vi "Remote Client Metrics subVI.vi"(9 "Message size":i32=1000000, 10 "Number of Messages":i32=20, 11 "RC Type":T1=enum."STM") -> (0 "<time/message (ms)>":i32=210, 1 "bytes/second":dbl=37611866.47860837, 2 "messages/second":dbl=4.701457451810062, 3 "<size>":i32=8000044)   [LabVIEW 2019]
uses:
  lvsrc/SMOs/RemoteControl/RemoteControl.lvclass
  lvsrc/SMOs/RemoteControl/Typedefs/RC Com Type--enum.ctl
panel:
  out "length":i32=8000004
  in  "stop":bool
  out "error out":errorcluster
  out "Data out":variant
  out "Command out":string="Command1"
  in  "Command":string="Command1"
  in  "address":string
  in  "Port":u16=6341
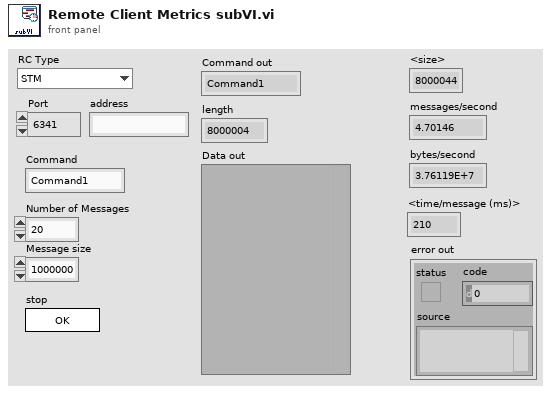
[diagram p1: front panel]
types:
  T1 = typedef "RemoteControl.lvclass/RC Com Type--enum.ctl" = enum16{"RC", "STM", "ZMQ"}
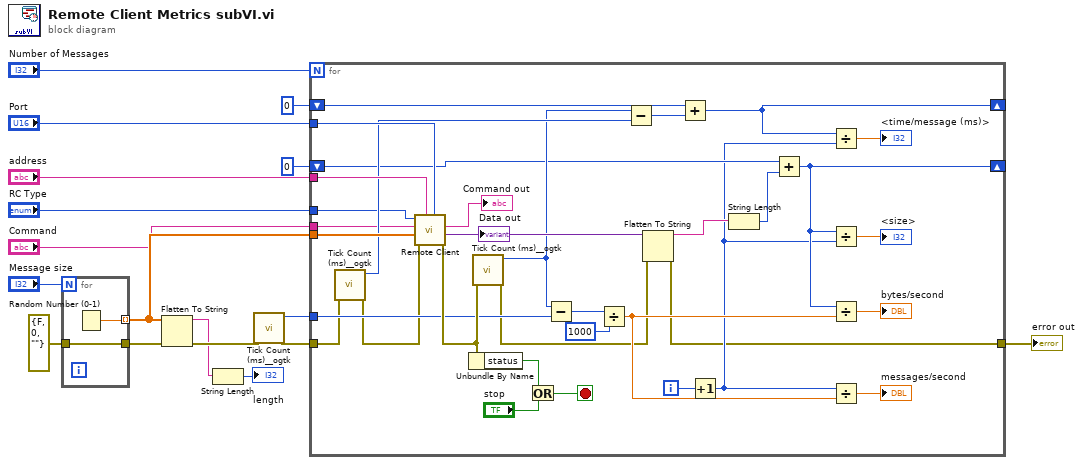
[diagram p0: block diagram]
diagram:
  n1 = for {
    N: "Message size" -> [_]
    tunnel: [w19] -> w10
    tunnel: errorcluster {"status"=FALSE, "code"=0, "source"=""} ("error in (no error)") -> [w19]
    tunnel: [w18] -> w2 mode=indexing
    n2 = Random Number (0-1)() -> (number: 0 to 1=w18:dbl)
  }
  n3 = Flatten To String(anything=w2, error in (no error)=w10) -> (data string=w7:string, error out=w9:errorcluster)  [unwired: 2 in, 1 out]
  n4 = String Length(string=w7) -> (length=→"length":i32)
  n5 = call <userlib>:"Tick Count (ms)__ogtk.vi"("error in (no error)"=w9) -> ("error out"=w14:errorcluster, "millisecond timer value"=w13:u32)  [unwired: 9 in]
  n6 = for {
    N: "Number of Messages" -> [_]
    tunnel: "Port" -> [w53]
    tunnel: [w22] -> w15
    tunnel: "address" -> [w52]
    tunnel: w14 -> [w35]
    tunnel: w13 -> [w46]
    tunnel: w2 -> [w38]
    shift-right: [w26] -> _
    shift-left: 0 -> [w29]
    shift-right: [w27] -> _
    shift-left: 0 -> [w28]
    tunnel: "Command" -> [w21]
    tunnel: "RC Type" -> [w20]
    i -> [w47]
    stop <- w37 stop-if-true
    n7 = call <userlib>:"Tick Count (ms)__ogtk.vi"("error in (no error)"=w35) -> ("error out"=w34:errorcluster, "millisecond timer value"=w33:u32)  [unwired: 9 in]
    n8 = call "Remote Client.vi"("Port"=w53, "address"=w52, "error in (no error)"=w34, "Data"=w38, "Command"=w21, "RC Type"=w20) -> ("error out"=w50:errorcluster, "Data out"=w42:variant, "Command out"=→"Command out":string)  [unwired: 2 in, 1 out]
    "Data out" <- w42
    n9 = Unbundle By Name(w50) -> ("status"=w48:bool)
    n10 = call <userlib>:"Tick Count (ms)__ogtk.vi"("error in (no error)"=w50) -> ("error out"=w23:errorcluster, "millisecond timer value"=w32:u32)  [unwired: 9 in]
    n11 = Or(x=w48, y="stop") -> (x .or. y?=w37:bool)
    n12 = Subtract(x=w32, y=w46) -> (x-y=w45:u32)
    n13 = Divide(x=w45, y=u32 1000) -> (x/y=w40:dbl)
    n14 = Subtract(x=w32, y=w33) -> (x-y=w31:u32)
    n15 = Flatten To String(anything=w42, error in (no error)=w23) -> (data string=w41:string, error out=w22:errorcluster)  [unwired: 2 in, 1 out]
    n16 = Add(x=w28, y=w31) -> (x+y=w27:u32)
    n17 = Increment(x=w47) -> (x+1=w25:i32)
    n18 = String Length(string=w41) -> (length=w36:i32)
    n19 = Add(x=w29, y=w36) -> (x+y=w26:i32)
    n20 = Divide(x=w27, y=w25) -> (x/y=→"<time/message (ms)>":dbl)
    n21 = Divide(x=w26, y=w25) -> (x/y=→"<size>":dbl)
    n22 = Divide(x=w26, y=w40) -> (x/y=→"bytes/second":dbl)
    n23 = Divide(x=w25, y=w40) -> (x/y=→"messages/second":dbl)
  }
  "error out" <- w15
